vi "InsertEntuse.vi"(9 "Entity":string, 11 "Date":string) -> ()   [LabVIEW 2012]
uses:
  <vilib>/addons/database/Connection.llb/DB Tools Open Connec (Path).vi
  <vilib>/addons/database/Connection.llb/Conn Execute.vi
  <vilib>/addons/database/Recordset.llb/Rec Fetch Recordset Data (R).vi
  <vilib>/addons/database/Recordset.llb/Rec Destroy - Connection.vi
  <vilib>/addons/database/_DB Variant To Data/Database Variant To Data.xnode
  <vilib>/addons/database/NI_Database_API.lvlib
panel:
  out "concatenated string":string
  out "recordset data":variant[][](array[variant])
  out "String":string
  out "array":string[][](array[string])
  out "error out":errorcluster
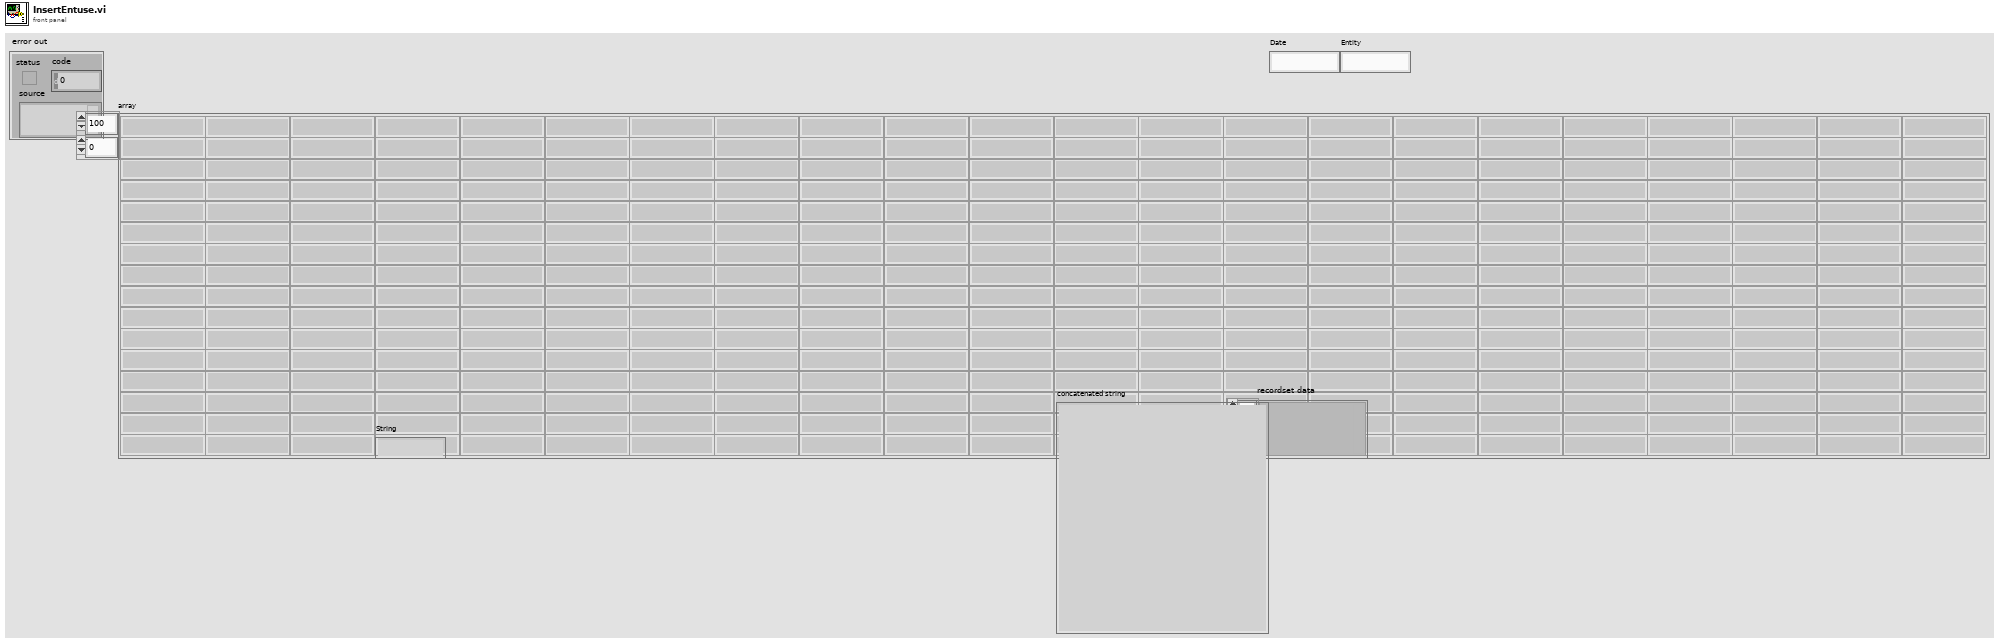
[diagram p1: front panel]
types:
  T1 = typedef "NI_Database_API.lvlib/Conn ObjectReference.ctl" = refnum<k1>
  T2 = typedef "NI_Database_API.lvlib/Rec ObjectReference.ctl" = refnum<k1>
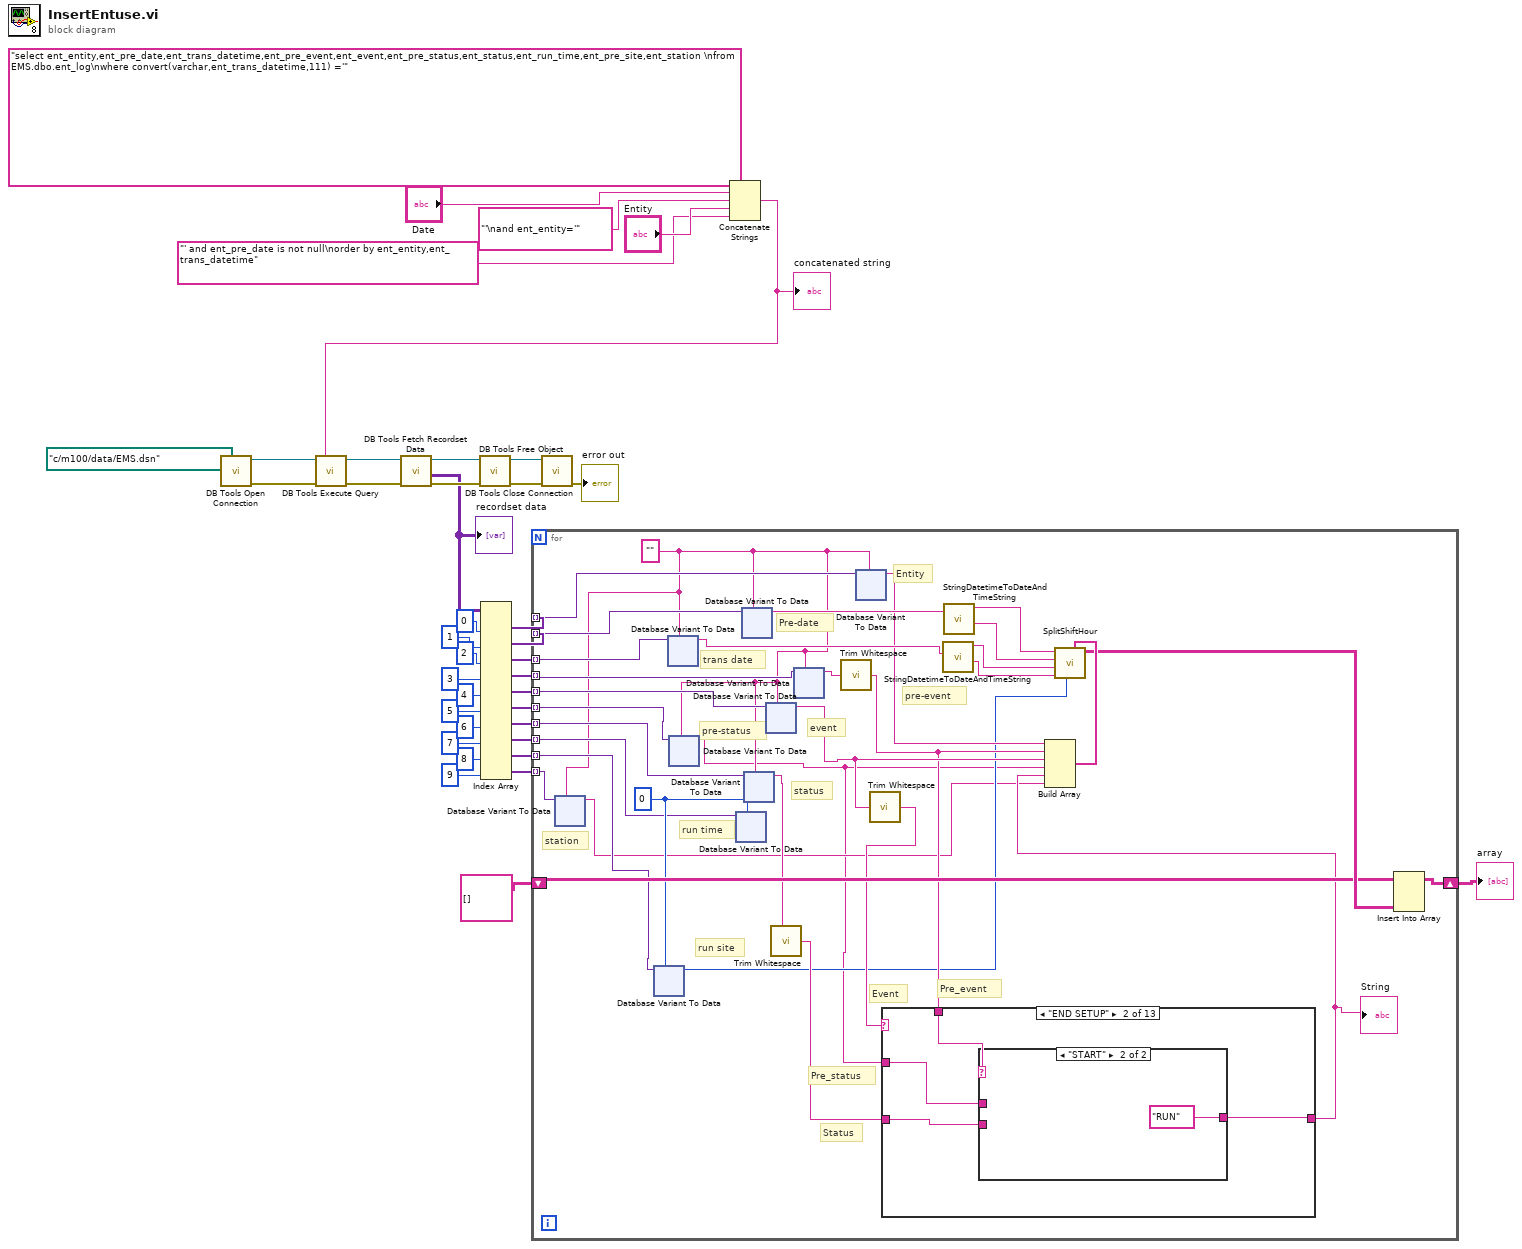
[diagram p0: block diagram]
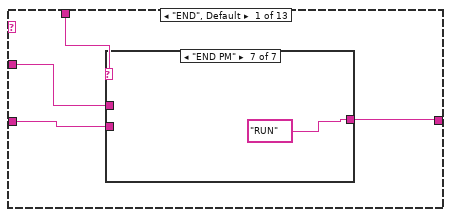
[diagram p2: hidden frame]
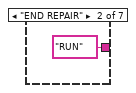
[diagram p4: hidden frame]
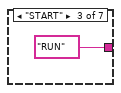
[diagram p5: hidden frame]
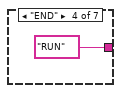
[diagram p6: hidden frame]
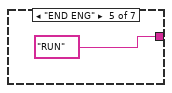
[diagram p7: hidden frame]
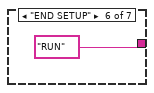
[diagram p8: hidden frame]
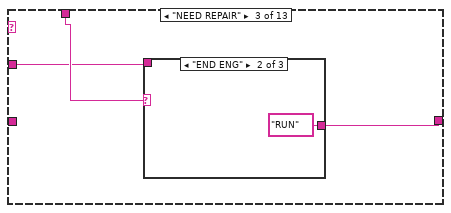
[diagram p10: hidden frame]
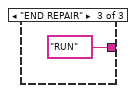
[diagram p12: hidden frame]
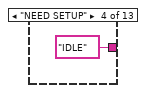
[diagram p13: hidden frame]
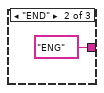
[diagram p15: hidden frame]
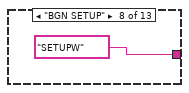
[diagram p20: hidden frame]
diagram:
  n1 = call-poly <vilib>:"DB Tools Open Connection.vi"("connection information"=path "c:/m100/data/EMS.dsn") -> ("error out"=w35:errorcluster, "connection reference"=w39:T1)  [unwired: 7 in]
  n2 = Concatenate Strings("select ent_entity,ent_pre_date,ent_trans_datetime,ent_pre_event,ent_event,ent_pre_status,ent_status,ent_run_time,ent_pre_site,ent_station \nfrom EMS.dbo.ent_log\nwhere convert(varchar,ent_trans_datetime,111) ='" ("string"), "Date", "'\nand ent_entity='" ("string"), "Entity", "' and ent_pre_date is not null\norder by ent_entity,ent_trans_datetime" ("string")) -> (w3:string)
  "concatenated string" <- w3
  n3 = call-poly <vilib>:"DB Tools Execute Query.vi"("error in (no error)"=w35, "SQL query"=w3, "connection reference"=w39) -> ("error out"=w34:errorcluster, "recordset reference"=w38:T2)  [unwired: 5 in]
  n4 = call-poly <vilib>:"DB Tools Fetch Recordset Data.vi"("error in (no error)"=w34, "recordset reference"=w38) -> ("error out"=w33:errorcluster, "recordset data"=w29:variant[][], "recordset reference out"=w37:T2)  [unwired: 3 in]
  "recordset data" <- w29
  n5 = call-poly <vilib>:"DB Tools Free Object.vi"("error in (no error)"=w33, "recordset reference"=w37) -> ("error out"=w32:errorcluster, "connection reference"=w36:T1)  [unwired: 8 in]
  n6 = Index Array(array=w29, index (col) #1=0 ("disabled index (col)"), index (col) #2=1 ("index (col)"), index (col) #3=2 ("index (col)"), index (col) #4=3 ("index (col)"), index (col) #5=4 ("index (col)"), index (col) #6=5 ("index (col)"), index (col) #7=6 ("index (col)"), index (col) #8=7 ("index (col)"), index (col) #9=8 ("index (col)"), index (col) #10=9 ("index (col)")) -> (element #1=w22:variant[], element #2=w21:variant[], element #3=w20:variant[], element #4=w19:variant[], element #5=w18:variant[], element #6=w17:variant[], element #7=w16:variant[], element #8=w13:variant[], element #9=w9:variant[], element #10=w1:variant[])  [unwired: 10 in]
  n7 = for {
    tunnel: w22 -> [w72] mode=indexing
    tunnel: w21 -> [w71] mode=indexing
    tunnel: w20 -> [w70] mode=indexing
    tunnel: w19 -> [w69] mode=indexing
    tunnel: w18 -> [w68] mode=indexing
    tunnel: w17 -> [w67] mode=indexing
    tunnel: w16 -> [w44] mode=indexing
    tunnel: w13 -> [w43] mode=indexing
    shift-right: [w57] -> w11
    shift-left: string[][] [] ("array") -> [w56]
    tunnel: w9 -> [w49] mode=indexing
    tunnel: w1 -> [w45] mode=indexing
    w48 = 0
    w42 = ""
    # "Status"
    # "Pre_status"
    # "Event"
    # "Pre_event"
    # "station"
    # "run site"
    # "run time"
    # "status"
    # "pre-status"
    # "event"
    # "pre-event"
    # "trans date"
    # "Pre-date"
    # "Entity"
    n8 = xnode "Database Variant To Data"("database variant"=w45, "type"=w42) -> ("data"=w41:string)  [unwired: 1 in, 1 out]
    n9 = xnode "Database Variant To Data"("database variant"=w49, "type"=w48) -> ("data"=w46:i32)  [unwired: 1 in, 1 out]
    n10 = xnode "Database Variant To Data"("database variant"=w70, "type"=w42) -> ("data"=w65:string)  [unwired: 1 in, 1 out]
    n11 = xnode "Database Variant To Data"("database variant"=w67, "type"=w42) -> ("data"=w40:string)  [unwired: 1 in, 1 out]
    n12 = xnode "Database Variant To Data"("database variant"=w43, "type"=w48) -> ()  [unwired: 1 in, 2 out]
    n13 = xnode "Database Variant To Data"("database variant"=w71, "type"=w42) -> ("data"=w66:string)  [unwired: 1 in, 1 out]
    n14 = xnode "Database Variant To Data"("database variant"=w44, "type"=w42) -> ("data"=w53:string)  [unwired: 1 in, 1 out]
    n15 = xnode "Database Variant To Data"("database variant"=w68, "type"=w42) -> ("data"=w55:string)  [unwired: 1 in, 1 out]
    n16 = call <vilib>:"Trim Whitespace.vi"("string"=w53) -> ("trimmed string"=w52:string)  [unwired: 1 in]
    n17 = xnode "Database Variant To Data"("database variant"=w69, "type"=w42) -> ("data"=w51:string)  [unwired: 1 in, 1 out]
    n18 = call <vilib>:"Trim Whitespace.vi"("string"=w51) -> ("trimmed string"=w50:string)  [unwired: 1 in]
    n19 = xnode "Database Variant To Data"("database variant"=w72, "type"=w42) -> ("data"=w60:string)  [unwired: 1 in, 1 out]
    n20 = call <vilib>:"Trim Whitespace.vi"("string"=w55) -> ("trimmed string"=w54:string)  [unwired: 1 in]
    n21 = case shown="\"END SETUP\"" w54 {
      tunnel: [w139 w150 w155 "IDLE" ("data") w161 w167 w169 "SETUPW" w175 w181 w189 w190 w197] -> w47
      tunnel: w52 -> [w138 w149 _ _ _ w167 w170 _ _ _ _ _ _]
      tunnel: w50 -> [w140 w151 w156 _ w163 _ w171 _ w177 w182 _ w192 w196]
      tunnel: w40 -> [w137 w148 w154 _ w162 _ w168 _ w176 w180 w189 w191 w198]
      frame "END", Default {
        n22 = case shown="\"END PM\"" w140 {
          tunnel: [w141 "RUN" ("data") "RUN" "RUN" "RUN" "RUN" "RUN"] -> w139
          tunnel: w138 -> [_ _ _ _ _ _ _]
          tunnel: w137 -> [w141 _ _ _ _ _ _]
          frame "False", Default {
          }
          frame "END REPAIR" {
          }
          frame "START" {
          }
          frame "END" {
          }
          frame "END ENG" {
          }
          frame "END SETUP" {
          }
          frame "END PM" {
          }
        }
      }
      frame "END SETUP" {
        n23 = case shown="\"START\"" w151 {
          tunnel: [w152 "RUN"] -> w150
          tunnel: w149 -> [_ _]
          tunnel: w148 -> [w152 _]
          frame "BGN SETUP", Default {
          }
          frame "START" {
          }
        }
      }
      frame "NEED REPAIR" {
        n24 = case shown="\"END ENG\"" w156 {
          tunnel: [w157 "RUN" ("data") "RUN"] -> w155
          tunnel: w154 -> [w157 _ _]
          frame "False", Default {
          }
          frame "END ENG" {
          }
          frame "END REPAIR" {
          }
        }
      }
      frame "NEED SETUP" {
      }
      frame "END ENG" {
        n25 = case shown="\"False\", Default" w163 {
          tunnel: [w164 "ENG" ("data") w166] -> w161
          tunnel: w162 -> [w164 _ w166]
          frame "False", Default {
          }
          frame "END" {
          }
          frame "START" {
          }
        }
      }
      frame "IDLE" {
      }
      frame "BGN REPAIR" {
        n26 = case shown="\"START\"" w171 {
          tunnel: w170 -> [_ _]
          tunnel: [w172 w173] -> w169
          tunnel: w168 -> [w172 w173]
          frame "False", Default {
          }
          frame "START" {
          }
        }
      }
      frame "BGN SETUP" {
      }
      frame "END REPAIR" {
        n27 = case shown="\"False\", Default" w177 {
          tunnel: [w178 "REPAIR" ("data")] -> w175
          tunnel: w176 -> [w178 _]
          frame "False", Default {
          }
          frame "END" {
          }
        }
      }
      frame "START" {
        n28 = case shown="\"END PM\"" w182 {
          tunnel: [w183 "ENG" ("trimmed string") "IDLE" "IDLE" "IDLE" "SETUP"] -> w181
          tunnel: w180 -> [w183 _ _ _ _ _]
          frame "False", Default {
          }
          frame "BGN ENG" {
          }
          frame "END" {
          }
          frame "END PM" {
          }
          frame "END ENG" {
          }
          frame "BGN SETUP" {
          }
        }
      }
      frame "BGN ENG" {
      }
      frame "BGN PM" {
        n29 = case shown="\"END REPAIR\"" w192 {
          tunnel: w191 -> [w193 _ _]
          tunnel: [w193 "RUN" ("data") "RUN" ("data")] -> w190
          frame "False", Default {
          }
          frame "END REPAIR" {
          }
          frame "END ENG" {
          }
        }
      }
      frame "END PM" {
        n30 = case shown="\"START\"" w196 {
          tunnel: w198 -> [w199 _]
          tunnel: [w199 "PM" ("data")] -> w197
          frame "False", Default {
          }
          frame "START" {
          }
        }
      }
    }
    "String" <- w47
    n31 = call "StringDatetimeToDateAndTimeString.vi"("String"=w65) -> ("Time String"=w61:string, "Date String"=w62:string)  [unwired: 8 in, 1 out]
    n32 = call "StringDatetimeToDateAndTimeString.vi"("String"=w66) -> ("Time String"=w63:string, "Date String"=w64:string)  [unwired: 8 in, 1 out]
    n33 = Build Array(w60, w50, w55, w40, w47, w41) -> (w59:string[])
    n34 = call "SplitShiftHour.vi"("BasicData"=w59, "Site"=w46, "EndTime 2"=w61, "date string"=w62, "BegTime"=w63, "BegDate"=w64) -> ("array"=w58:string[][])  [unwired: 5 in]
    n35 = Insert Into Array(array=w56, new element=w58) -> (w57:string[][])  [unwired: 2 in]
  }
  "array" <- w11
  n36 = call <vilib>:"DB Tools Close Connection.vi"("error in (no error)"=w32, "connection reference"=w36) -> ("error out"=→"error out":errorcluster)  [unwired: 5 in]
